vi "Renishaw-XL80_GetMatCompFactor.vi"(8 "error in (no error)":errorcluster, 11 "Renishaw-XL80 in":refnum<class "Renishaw-XL80.lvclass">) -> (0 "error out":errorcluster, 2 "MatCompFactor":dbl, 3 "Renishaw-XL80 out":refnum<class "Renishaw-XL80.lvclass">)   [LabVIEW 2024, in "Renishaw-XL80.lvclass"]
doc: "Reading this property retrieves the current material compensation factor.\n\nDefinition\nHRESULTget_MatCompFactor( [out, retval] double* pVal);\nParameters\npVal\nA variable that will be set to the current material compensation factor.\n\nComments\nReading this property will always retrieve the current material compensation factor. The material compensation factor is a factor which when multiplied by the raw laser measurement will compensate the reading for thermal growth of the material, thereby estimating the reading that would be obtained if the material temperature had been 20°C. Note that MatCompFactor is a value very close to 1.00. For example if the expansion coefficient is set to 10ppm/°C and the current material temperature is 25°C then MatCompFactor will be 0.9999\n\nThe property will normally return an HRESULT of S_OK. However, it will return E_POINTER if the client supplies a null pointer for pVal."
uses:
  Renishaw-XL80.lvclass
  Renishaw-XL80.lvclass/Renishaw-XL80.ctl
  D:/A.C.M/Example CSharp_64/bin/Debug/Interop.DX10SDKADAPTORLib.dll
  Example CSharp_64/bin/Debug/Interop.DX10SDKADAPTORLib.dll
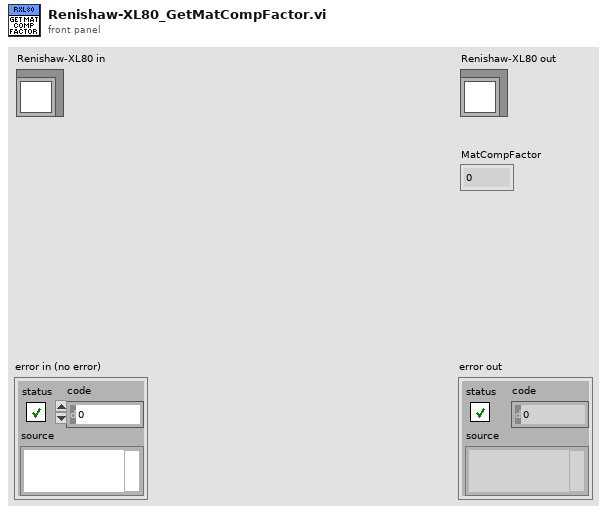
[diagram p1: front panel]
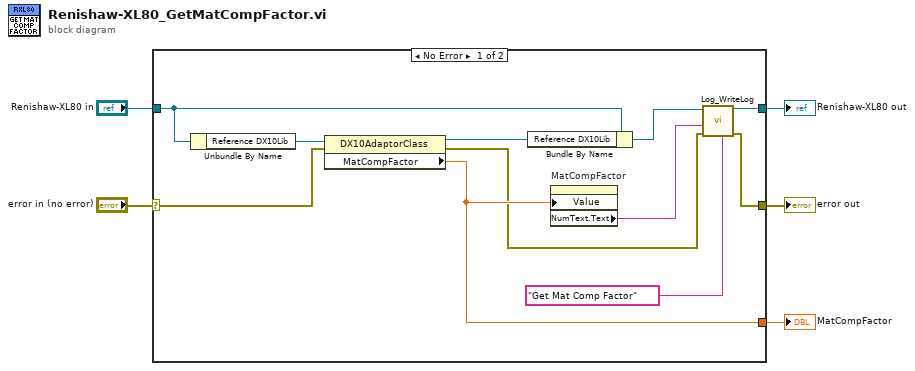
[diagram p0: block diagram]
diagram:
  n1 = case shown="No Error" "error in (no error)" {
    selector: "error in (no error)" -> [w13 w18]
    tunnel: [w11 w18] -> w4
    tunnel: [w12 w17] -> w2
    tunnel: "Renishaw-XL80 in" -> [w14 w17]
    tunnel: [w10 _] -> w1
    frame No Error {
      n2 = Unbundle By Name(w14) -> ("Reference DX10Lib"=w16:refnum<k24>)
      n3 = property class="DX10AdaptorClass"(reference=w16, error in=w13) -> (reference out=w15:refnum<k24>, error out=w6:errorcluster, "MatCompFactor"=w10:dbl)
      n4 = Bundle By Name(cluster=w14, "Reference DX10Lib"=w15) -> (w9:refnum<class "Renishaw-XL80.lvclass">)
      n5 = property on="MatCompFactor" class="DigNum (strict)"("Value"=w10) -> ("NumText.Text"=w8:string)  [unwired: 2 in, 2 out]
      n6 = call-dynamic "Log_WriteLog.vi"("Additional text"="Get Mat Comp Factor", "error in (no error)"=w6, "Response"=w8, "Log in"=w9) -> ("error out"=w11:errorcluster, "Log out"=w12:refnum<class "Renishaw-XL80.lvclass">)  [unwired: 6 in]
    }
    frame Error {
    }
  }
  "error out" <- w4
  "Renishaw-XL80 out" <- w2
  "MatCompFactor" <- w1
